vi "Digital Output - N Channel - N Sample.vi"() -> ()   [LabVIEW 2019]
uses:
  <vilib>/myRIO/Instrument Drivers/Onboard IO/DO Block/typedefs/DO Block Reference.ctl
  <vilib>/myRIO/Common/Instrument Driver Framework/Utilities/typedefs/myRIO Generic Hardware Reference.ctl
  <vilib>/myRIO/Common/Instrument Driver Framework/Utilities/typedefs/Hardware Version Enum.ctl
  <vilib>/myRIO/Common/Instrument Driver Framework/Utilities/typedefs/myRIO v1.0 Reference.ctl
  <vilib>/myRIO/Common/Instrument Driver Framework/Utilities/typedefs/Generic FPGA Reference.ctl
  <vilib>/myRIO/Common/Instrument Driver Framework/myRIO v1.0/DO Block/typedefs/DO Block Channels List.ctl
  <vilib>/myRIO/Common/Instrument Driver Framework/myRIO v1.0/DO Block/typedefs/DO Block Channels Enum.ctl
  <vilib>/userdefined/High Color/nirio_resource_hc.ctl
  <vilib>/myRIO/Common/Instrument Driver Framework/Utilities/vis/Is FPGA Ref Available.vi
  <vilib>/myRIO/Common/Instrument Driver Framework/ELVIS III v1.0/DO Block/vis/ELVIS III v1.1 Open DO (N Samples).vi
  <vilib>/myRIO/Instrument Drivers/Onboard IO/DO Block/vis/Write.vi
  <vilib>/myRIO/Common/Instrument Driver Framework/Utilities/vis/Validate Channels.vi
  <vilib>/myRIO/Common/Instrument Driver Framework/ELVIS III v1.0/Resource Manager/vis/ELVIS III v1.0 Check For Different Banks.vi
  <vilib>/myRIO/Common/Instrument Driver Framework/ELVIS III v1.0/DO Block/vis/ELVIS III v1.0 DO Block Write.vi
  <vilib>/myRIO/Common/Instrument Driver Framework/myRIO v1.0/UART/vis/myRIO v1.0 Close UART.vi
  <vilib>/myRIO/Common/Instrument Driver Framework/Utilities/vis/Sample Rate To Ticks.vi
  <vilib>/Waveform/DWDTOps.llb/Digital Pattern Generator (Ramp).vi
  <vilib>/Waveform/DWDTOps.llb/DWDT Digital to Boolean Array.vi
  <vilib>/myRIO/Instrument Drivers/Utilities/vis/Reset Index.vi
  <vilib>/Utility/VariantDataType/GetNumericInfo.vi
  <vilib>/Utility/error.llb/Error Cluster From Error Code.vi
  <vilib>/myRIO/Common/Instrument Driver Framework/ELVIS III v1.0/ELVIS III v1.1 Open.vi
  <vilib>/myRIO/Common/Instrument Driver Framework/ELVIS III v1.0/DO Block/vis/ELVIS III v1.0 Reserve DO Block.vi
  <vilib>/myRIO/Common/Instrument Driver Framework/ELVIS III v1.0/Resource Manager/vis/ELVIS III v1.0 Configure DMAs.vi
  <vilib>/myRIO/Common/Instrument Driver Framework/ELVIS III v1.0/Resource Manager/vis/ELVIS III v1.0 Open Writing DMA.vi
  <vilib>/myRIO/Common/Instrument Driver Framework/myRIO v1.0/myRIO v1.0 Close.vi
  <vilib>/myRIO/Common/Instrument Driver Framework/myRIO v1.0/Resource Manager/vis/myRIO v1.0 Block Write Configuration.vi
  <vilib>/myRIO/Common/Instrument Driver Framework/ELVIS III v1.0/DO Block/vis/ELVIS III v1.0 DO Build Bank Data.vi
  <vilib>/myRIO/Common/Instrument Driver Framework/ELVIS III v1.0/DO Block/vis/ELVIS III v1.0 DO Enqueue Data.vi
  <vilib>/myRIO/Common/Instrument Driver Framework/Utilities/vis/FPGA Ref Manager.vi
  <vilib>/myRIO/Common/Instrument Driver Framework/ELVIS III v1.0/ELVIS III v1.0 Reset FPGA.vi
  <vilib>/myRIO/Common/Instrument Driver Framework/myRIO v1.0/IRQ/vis/myRIO v1.0 IRQ Info FGV.vi
  <vilib>/myRIO/Common/Instrument Driver Framework/myRIO v1.0/IRQ/vis/myRIO v1.0 Timer IRQ Info FGV.vi
  <vilib>/myRIO/Common/Instrument Driver Framework/myRIO v1.0/IRQ/vis/myRIO v1.0 ISR Agent.vi
  <vilib>/myRIO/Common/Instrument Driver Framework/myRIO v1.0/Resource Manager/vis/myRIO v1.0 Block Write Resource Manager.vi
  <vilib>/myRIO/Express VI/Onboard IO/DO/DO Express VI.xnode
  <vilib>/myRIO/Instrument Drivers/Onboard IO/DO Block/vis/myRIO DO N Samples Open.xnode
  <vilib>/myRIO/Instrument Drivers/Utilities/Utilities.lvlib
  <vilib>/myRIO/Instrument Drivers/Onboard IO/DO Block/DO Block.lvlib
panel:
  in  "Stop":bool
  out "Digital Waveform Graph":digitalwaveform(graph)
  in  "Generate Ramp":bool
  # "ELVIS III Control IO"
  # "数字输出N通道"
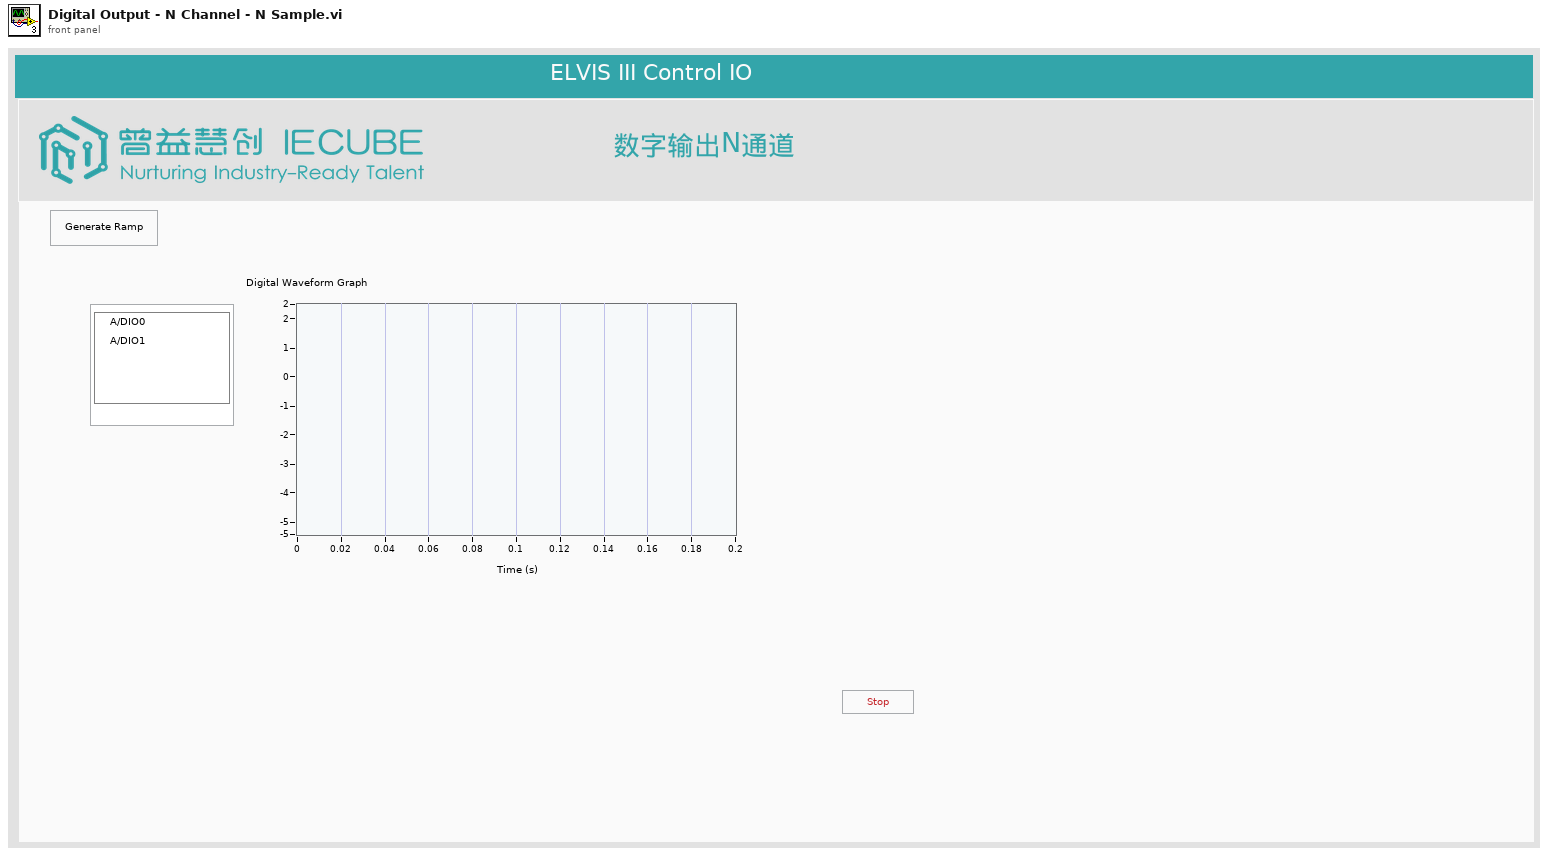
[diagram p1: front panel]
types:
  T1 = typedef "DO Block.lvlib/DO Block Reference.ctl" = cluster{"myRIO Reference":T2, "DO (N Samples) Channels List":T6}
  T2 = typedef "myRIO Generic Hardware Reference.ctl" = cluster{"myRIO Model":T3, "myRIO Hardware Reference":T4}
  T3 = typedef "Hardware Version Enum.ctl" = enum16{"Unknown", "myRIO-1900", "myRIO-1950", "roboRIO", "NI ELVIS RIO CM", "ELVIS III"}
  T4 = typedef "myRIO v1.0 Reference.ctl" = cluster{"Generic FPGA Reference":T5, "Allow multiple opens":bool}
  T5 = typedef "Generic FPGA Reference.ctl" = refnum<k20>
  T6 = typedef "DO Block Channels List.ctl" = T7[]
  T7 = typedef "DO Block Channels Enum.ctl" = enum16{"Not Connected", "A/DO0 (N Samples)", "A/DO1 (N Samples)", "A/DO2 (N Samples)", "A/DO3 (N Samples)", "A/DO4 (N Samples)", "A/DO5 (N Samples)", "A/DO6 (N Samples)", "A/DO7 (N Samples)", "A/DO8 (N Samples)", "A/DO9 (N Samples)", "A/DO10 (N Samples)", "A/DO11 (N Samples)", "A/DO12 (N Samples)", "A/DO13 (N Samples)", "A/DO14 (N Samples)", "A/DO15 (N Samples)", "A/DO16 (N Samples)", "A/DO17 (N Samples)", "A/DO18 (N Samples)", "A/DO19 (N Samples)", "B/DO0 (N Samples)", "B/DO1 (N Samples)", "B/DO2 (N Samples)", "B/DO3 (N Samples)", "B/DO4 (N Samples)", "B/DO5 (N Samples)", "B/DO6 (N Samples)", "B/DO7 (N Samples)", "B/DO8 (N Samples)", "B/DO9 (N Samples)", "B/DO10 (N Samples)", "B/DO11 (N Samples)", "B/DO12 (N Samples)", "B/DO13 (N Samples)", "B/DO14 (N Samples)", "B/DO15 (N Samples)", "B/DO16 (N Samples)", "B/DO17 (N Samples)", "B/DO18 (N Samples)", "B/DO19 (N Samples)"}
  T8 = typedef "nirio_resource_hc.ctl" = tag
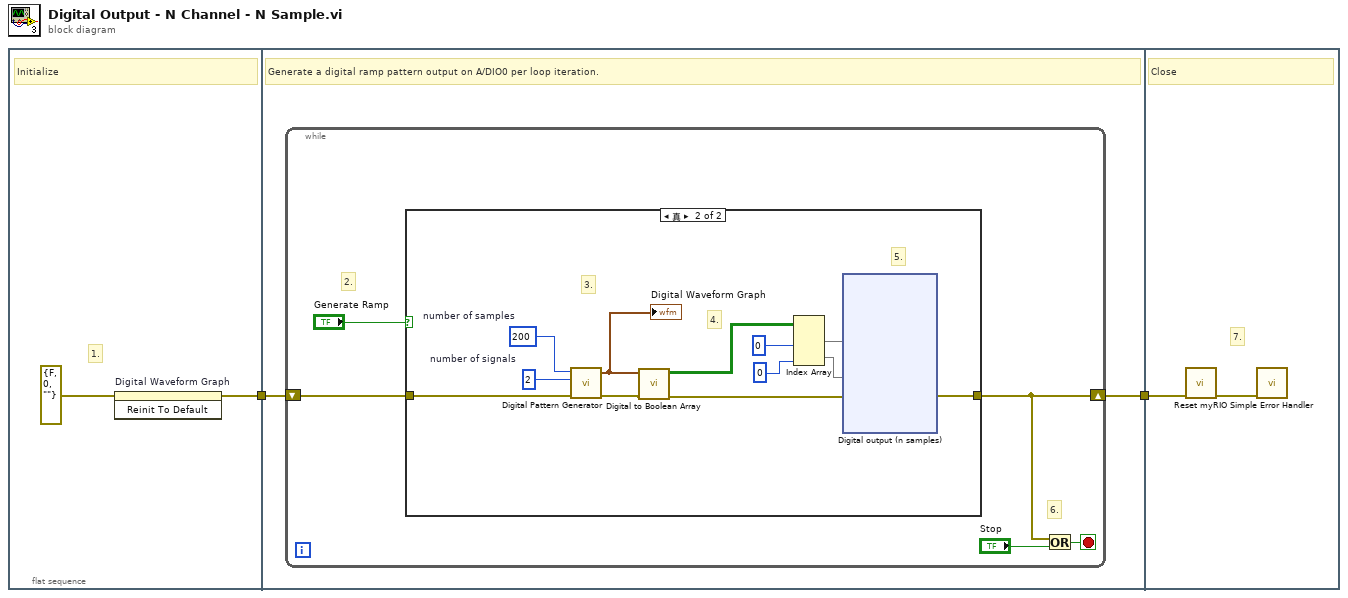
[diagram p0: block diagram]
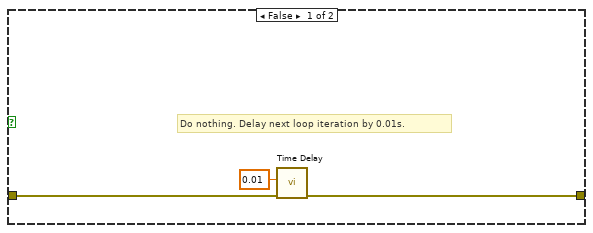
[diagram p2: hidden frame]
diagram:
  n1 = flat-sequence {
    tunnel: [w3] -> w2
    tunnel: [w6] -> w1
    tunnel: w2 -> [w5]
    tunnel: w1 -> [w76]
    frame #0 {
      # "1."
      # "Initialize"
      n2 = invoke on="Digital Waveform Graph" class="DigitalGraph (strict)" method="Reinit To Default"(error in=errorcluster {"status"=FALSE, "code"=0, "source"=""} ("Error In")) -> (error out=w3:errorcluster)  [unwired: 2 in, 2 out]
    }
    frame #1 {
      # "Generate a digital ramp pattern output on A/DIO0 per loop iteration."
      n3 = while {
        shift-right: [w9] -> w6
        shift-left: w5 -> [w8]
        stop <- w11 stop-if-true
        # "6."
        # "2."
        n4 = case shown="真" "Generate Ramp" {
          tunnel: [w13 w26] -> w9
          tunnel: w8 -> [w12 w21]
          frame False {
            # "Do nothing. Delay next loop iteration by 0.01s."
            n5 = call "Time Delay"("error in (no error)"=w12, "Delay Time (s)"=0.01) -> ("error out"=w13:errorcluster)  [unwired: 9 in]
          }
          frame True {
            w17 = u32 200  # number of samples
            w23 = u32 2  # number of signals
            # "5."
            # "4."
            # "3."
            n6 = call-poly <vilib>:"Digital Pattern Generator.vi"("error in (no error)"=w21, "number of signals"=w23, "number of samples"=w17) -> ("error out"=w18:errorcluster, "digital waveform"=w19:digitalwaveform)  [unwired: 7 in]
            "Digital Waveform Graph" <- w19
            n7 = call-poly <vilib>:"Digital to Boolean Array.vi"("error in (no error)"=w18, "digital waveform"=w19) -> ("error out"=w20:errorcluster, "boolean array"=w24:bool[][])  [unwired: 8 in]
            n8 = Index Array(array=w24, index (col) #1=0 ("disabled index (col)"), index (col) #2=0 ("索引 (列)")) -> (element #1=w22:bool[], element #2=w16:bool[])  [unwired: 2 in]
            n9 = xnode "Digital output (n samples)"("A/DO0 (N Samples)"=w22, "A/DO1 (N Samples)"=w16, "error in (no error)"=w20) -> ("error out"=w26:errorcluster)
          }
        }
        n10 = Or(x=w9, y="Stop") -> (x .or. y?=w11:bool)
      }
    }
    frame #2 {
      # "7."
      # "Close"
      n11 = call <vilib>:"Reset myRIO.vi"("error in (no error)"=w76) -> ("error out"=w75:errorcluster)  [unwired: 10 in]
      n12 = call <vilib>:"Simple Error Handler.vi"("error in (no error)"=w75) -> ()  [unwired: 4 in, 5 out]
    }
  }
